vi "GlobalStopGetBeamDiagnostics.vi"() -> ()   [LabVIEW 2013]
panel:
  in  "Stop Beam Diagnostic":bool
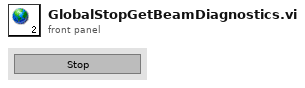
[diagram p1: front panel]
diagram:
